vi "log_table_first_row_in_push_down_rest.vi"(6 "String":string, 7 "tableIndx":i32 caption="Which Log Table", 8 "colIndx":i32 caption="Which Col Index", 9 "insertRow":i32, 10 "pass8thRow":bool, 11 "logTable in":string[][][](array[string])) -> (3 "logTable out":string[][][](array[string]))   [LabVIEW 2013]
panel:
  out "logTableOutNew":string[][](array[string])
  out "logTableOut":string[][](array[string])
  out "logTableIn":string[][](array[string])
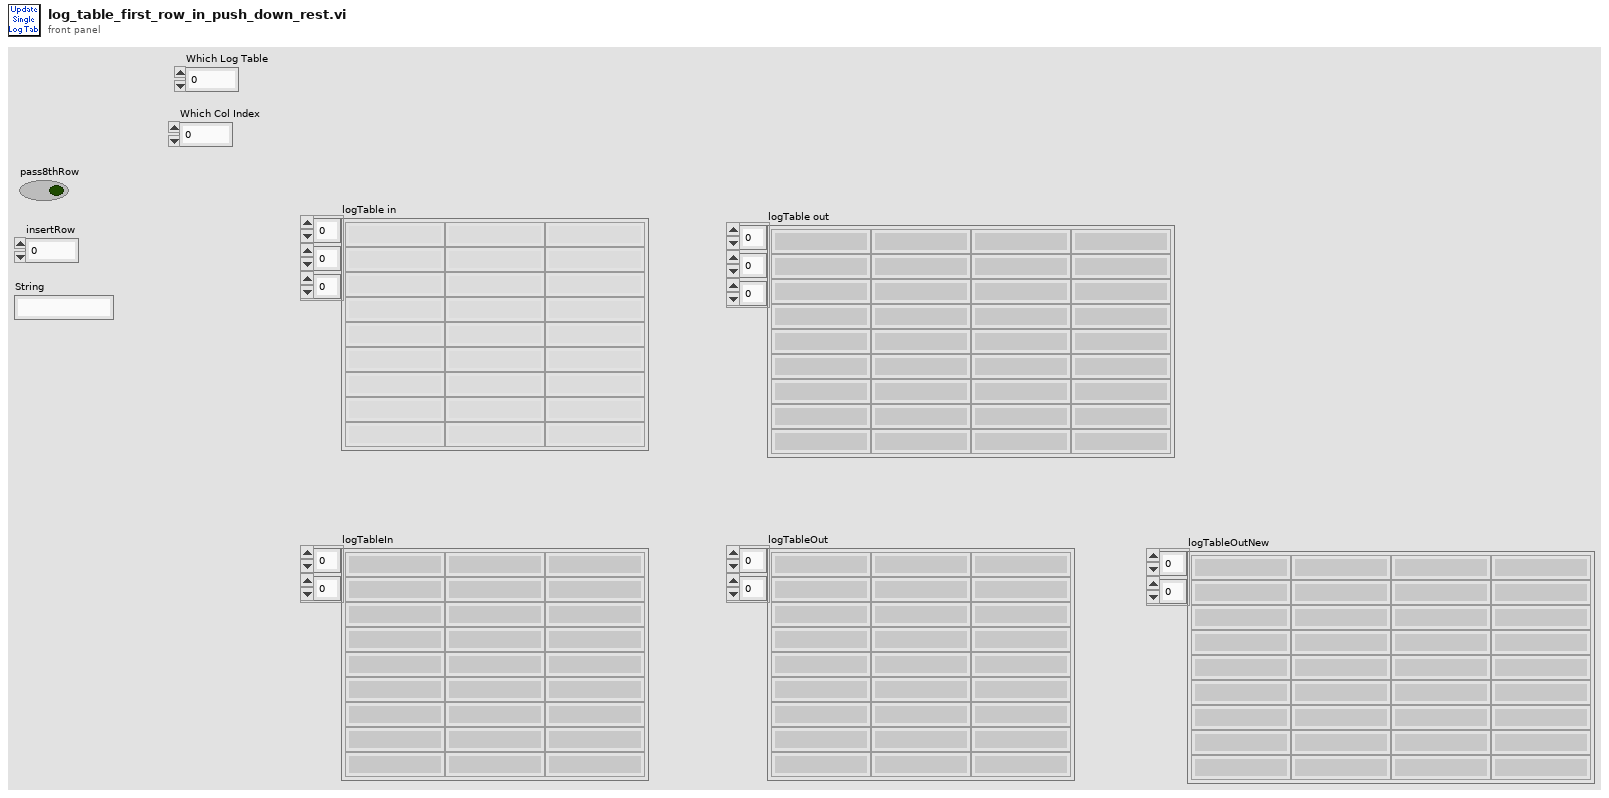
[diagram p1: front panel]
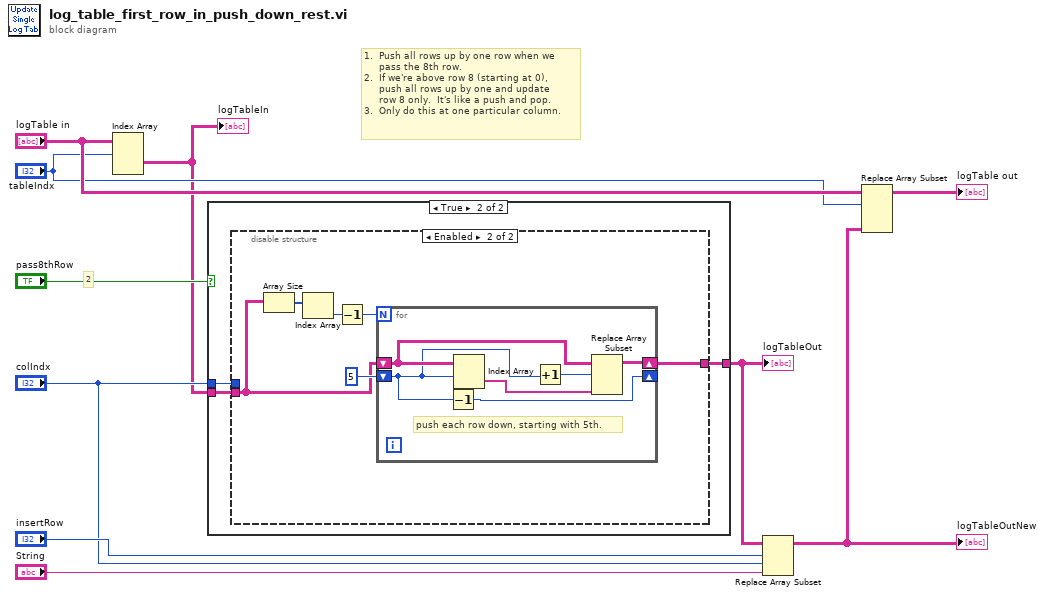
[diagram p0: block diagram]
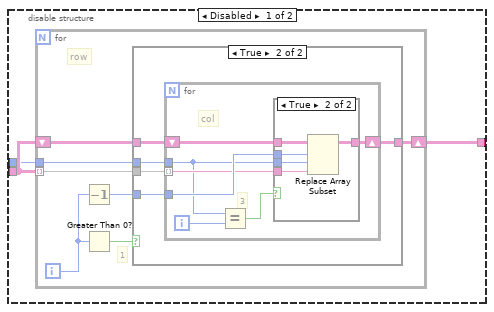
[diagram p3: hidden frame]
diagram:
  # "2"
  # "1.  Push all rows up by one row when we\n     pass the 8th row.\n2.  If we're above row 8 (starting at 0),\n     push all rows up by one and update\n     row 8 only.  It's like a push and pop.\n3.  Only do this at one particular column."
  n1 = Index Array(array="logTable in", index (dim 0)="tableIndx") -> (element=w1:string[][])  [unwired: 2 in]
  "logTableIn" <- w1
  n2 = case shown="True" "pass8thRow" {
    tunnel: w1 -> [w11 w14]
    tunnel: [w11 w13] -> w6
    tunnel: "colIndx" -> [_ w12]
    frame False {
    }
    frame True {
      n3 = disable-structure shown="Enabled" {
        disable-tunnel: w14 -> [w17 w45]
        disable-tunnel: [w16 w44] -> w13
        disable-tunnel: w12 -> [w15 _]
        frame Disabled {
          n4 = for {
            tunnel: w17 -> [w23] mode=indexing
            shift-right: [w22] -> w16
            shift-left: w17 -> [w24]
            tunnel: w15 -> [w21]
            i -> [w20]
            # "1"
            # "row"
            n5 = Decrement(x=w20) -> (x-1=w18:i32)
            n6 = Greater Than 0?(x=w20) -> (x > 0?=w19:bool)
            n7 = case shown="True" w19 {
              tunnel: w24 -> [w25 w30]
              tunnel: w23 -> [_ w29]
              tunnel: [w25 w28] -> w22
              tunnel: w21 -> [_ w27]
              tunnel: w18 -> [_ w26]
              frame False {
              }
              frame True {
                n8 = for {
                  tunnel: w29 -> [w33] mode=indexing
                  tunnel: w27 -> [w32]
                  shift-right: [w36] -> w28
                  shift-left: w30 -> [w37]
                  tunnel: w26 -> [w34]
                  i -> [w35]
                  # "3"
                  # "col"
                  n9 = Equal?(x=w32, y=w35) -> (x = y?=w31:bool)
                  n10 = case shown="True" w31 {
                    tunnel: w37 -> [w38 w43]
                    tunnel: [w38 w42] -> w36
                    tunnel: w34 -> [_ w41]
                    tunnel: w33 -> [_ w40]
                    tunnel: w32 -> [_ w39]
                    frame False {
                    }
                    frame True {
                      n11 = Replace Array Subset(array=w43, new element=w40, index (row)=w41, index (col)=w39) -> (w42:string[][])
                    }
                  }
                }
              }
            }
          }
        }
        frame Enabled {
          n12 = Array Size(array=w45) -> (size(s)=w47:i32[])
          n13 = Index Array(array=w47) -> (element=w48:i32)  [unwired: 1 in]
          n14 = Decrement(x=w48) -> (x-1=w49:i32)
          n15 = for {
            N: w49 -> [_]
            shift-right: [w52] -> w44
            shift-left: w45 -> [w55]
            shift-right: [w50] -> _
            shift-left: 5 ("index (row)") -> [w51]
            # "push each row down, starting with 5th."
            n16 = Decrement(x=w51) -> (x-1=w50:i32)
            n17 = Index Array(array=w55, index (row)=w51) -> (element=w53:string[])  [unwired: 1 in]
            n18 = Increment(x=w51) -> (x+1=w54:i32)
            n19 = Replace Array Subset(array=w55, new element=w53, index (row)=w54) -> (w52:string[][])  [unwired: 1 in]
          }
        }
      }
    }
  }
  "logTableOut" <- w6
  n20 = Replace Array Subset(array=w6, new element="String", index (row)="insertRow", index (col)="colIndx") -> (w5:string[][])
  "logTableOutNew" <- w5
  n21 = Replace Array Subset(array="logTable in", new element=w5, index (dim 0)="tableIndx") -> (→"logTable out":string[][][])  [unwired: 2 in]
